vi "server.vi"() -> ()   [LabVIEW 2021]
uses:
  <vilib>/Utility/file.llb/Read Delimited Spreadsheet (string).vi
  <vilib>/Utility/file.llb/Write Delimited Spreadsheet (string).vi
  <vilib>/regexp/Match Regular Expression.xnode
panel:
  out "reg-save-error":errorcluster
  out "log-save-error":errorcluster
  out "wash-fp":path
  out "user-fp":path
  out "log-error":errorcluster
  out "reg-error":errorcluster
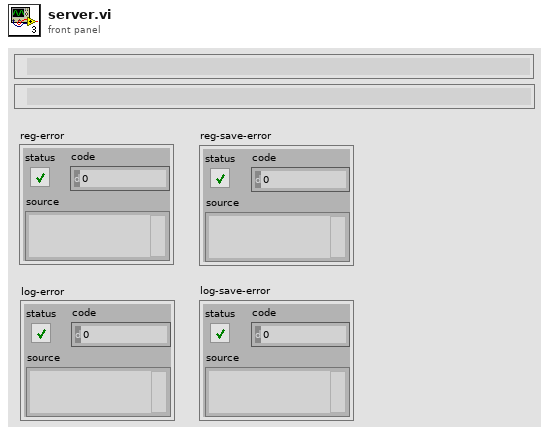
[diagram p1: front panel]
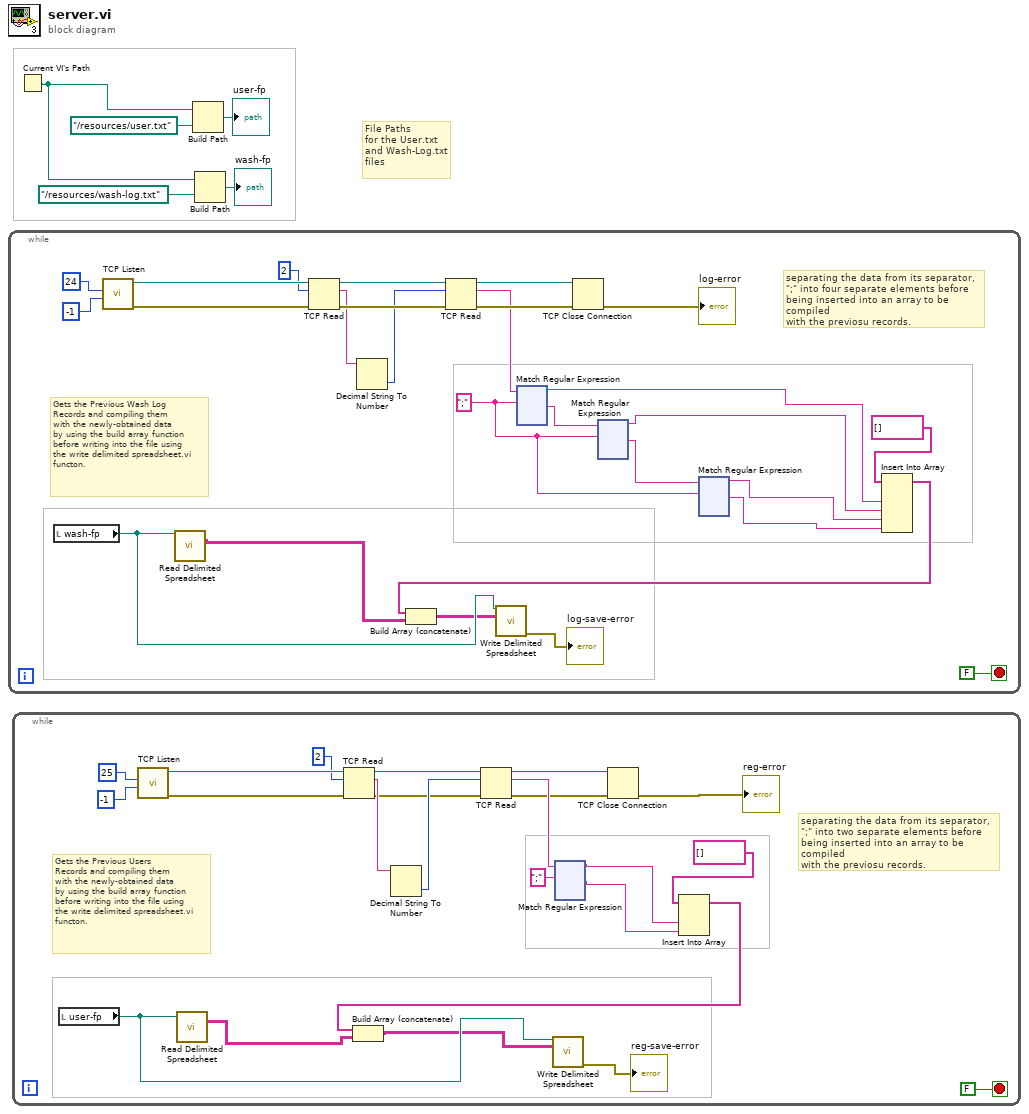
[diagram p0: block diagram]
diagram:
  # "File Paths\nfor the User.txt \nand Wash-Log.txt\nfiles"
  n1 = while {
    stop <- FALSE stop-if-true
    w16 = ";" ("regular expression")
    # "separating the data from its separator,\n\";\" into four separate elements before\nbeing inserted into an array to be compiled\nwith the previosu records."
    # "Gets the Previous Wash Log\nRecords and compiling them\nwith the newly-obtained data\nby using the build array function\nbefore writing into the file using\nthe write delimited spreadsheet.vi\nfuncton."
    n2 = local read "wash-fp"() -> (w10:path)
    n3 = call <vilib>:"TCP Listen.vi"("timeout ms (wait forever: -1)"=-1, "port"=u16 24) -> ("error out"=w24:errorcluster, "connection ID"=w29:refnum<k5>)  [unwired: 5 in, 3 out]
    n4 = call-poly <vilib>:"Read Delimited Spreadsheet.vi"("file path (dialog if empty)"=w10) -> ("all rows"=w11:string[][])  [unwired: 9 in, 5 out]
    n5 = TCP Read(connection ID=w29, bytes to read=2, error in (no error)=w24) -> (connection ID out=w28:refnum<k5>, data out=w21:string, error out=w25:errorcluster)  [unwired: 2 in]
    n6 = Decimal String To Number(string=w21) -> (number=w20:i32)  [unwired: 2 in, 1 out]
    n7 = TCP Read(connection ID=w28, bytes to read=w20, error in (no error)=w25) -> (connection ID out=w27:refnum<k5>, data out=w19:string, error out=w26:errorcluster)  [unwired: 2 in]
    n8 = xnode "Match Regular Expression"("input string"=w19, "regular expression"=w16) -> ("before match"=w15:string, "after match"=w18:string)  [unwired: 4 in, 3 out]
    n9 = TCP Close Connection(connection ID=w27, error in (no error)=w26) -> (error out=→"log-error":errorcluster)  [unwired: 1 in, 1 out]
    n10 = xnode "Match Regular Expression"("input string"=w18, "regular expression"=w16) -> ("before match"=w14:string, "after match"=w17:string)  [unwired: 4 in, 3 out]
    n11 = xnode "Match Regular Expression"("input string"=w17, "regular expression"=w16) -> ("before match"=w13:string, "after match"=w12:string)  [unwired: 4 in, 3 out]
    n12 = Insert Into Array "Insert Into Array"(array=string[] [], new element #1=w15, new element #2=w14, new element #3=w13, new element #4=w12) -> (w8:string[])  [unwired: 1 in]
    n13 = Build Array (concatenate) "Build Array"(w8, w11) -> (w7:string[][])
    n14 = call-poly <vilib>:"Write Delimited Spreadsheet.vi"("file path (dialog if empty)"=w10, "2D data"=w7) -> ("error out"=→"log-save-error":errorcluster)  [unwired: 12 in, 1 out]
  }
  n15 = while {
    stop <- FALSE stop-if-true
    # "Gets the Previous Users\nRecords and compiling them\nwith the newly-obtained data\nby using the build array function\nbefore writing into the file using\nthe write delimited spreadsheet.vi\nfuncton."
    # "separating the data from its separator,\n\";\" into two separate elements before\nbeing inserted into an array to be compiled\nwith the previosu records."
    n16 = local read "user-fp"() -> (w386:path)
    n17 = call <vilib>:"TCP Listen.vi"("timeout ms (wait forever: -1)"=-1, "port"=u16 25) -> ("error out"=w402:errorcluster, "connection ID"=w397:refnum<k5>)  [unwired: 5 in, 3 out]
    n18 = call-poly <vilib>:"Read Delimited Spreadsheet.vi"("file path (dialog if empty)"=w386) -> ("all rows"=w388:string[][])  [unwired: 9 in, 5 out]
    n19 = TCP Read(connection ID=w397, bytes to read=2, error in (no error)=w402) -> (connection ID out=w398:refnum<k5>, data out=w404:string, error out=w401:errorcluster)  [unwired: 2 in]
    n20 = Decimal String To Number(string=w404) -> (number=w405:i32)  [unwired: 2 in, 1 out]
    n21 = TCP Read(connection ID=w398, bytes to read=w405, error in (no error)=w401) -> (connection ID out=w399:refnum<k5>, data out=w406:string, error out=w400:errorcluster)  [unwired: 2 in]
    n22 = xnode "Match Regular Expression"("input string"=w406, "regular expression"=";") -> ("before match"=w391:string, "after match"=w390:string)  [unwired: 4 in, 3 out]
    n23 = TCP Close Connection(connection ID=w399, error in (no error)=w400) -> (error out=→"reg-error":errorcluster)  [unwired: 1 in, 1 out]
    n24 = Insert Into Array "Insert Into Array"(array=string[] [], new element #1=w391, new element #2=w390) -> (w387:string[])  [unwired: 1 in]
    n25 = Build Array (concatenate) "Build Array"(w387, w388) -> (w385:string[][])
    n26 = call-poly <vilib>:"Write Delimited Spreadsheet.vi"("file path (dialog if empty)"=w386, "2D data"=w385) -> ("error out"=→"reg-save-error":errorcluster)  [unwired: 12 in, 1 out]
  }
  n27 = Current VI's Path() -> (path=w3:path)
  n28 = Build Path(base path=w3, name or relative path=path "../resources/user.txt") -> (appended path=→"user-fp":path)
  n29 = Build Path(base path=w3, name or relative path=path "../resources/wash-log.txt") -> (appended path=→"wash-fp":path)
